vi "Write Dynamic.vi"(8 "error in (no error)":errorcluster, 10 "Dynamic data":dynamicdata(graph), 11 "tdms file":refnum<k34>) -> (0 "error out":errorcluster, 3 "tdms file out":refnum<k34>)   [LabVIEW 2015]
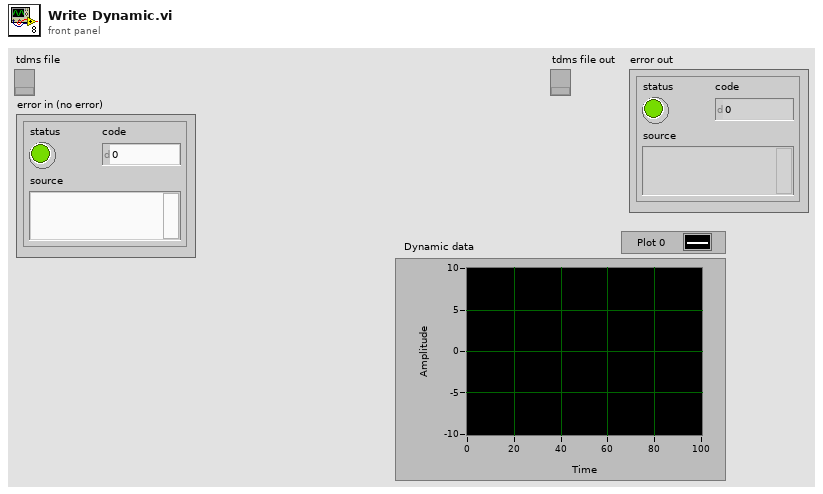
[diagram p1: front panel]
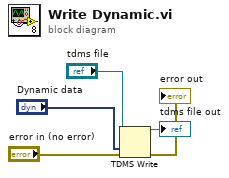
[diagram p0: block diagram]
diagram:
  n1 = TDMS Write(0:"tdms file", 9:"Dynamic data", 11:"error in (no error)") -> (4:→"tdms file out":refnum<k34>, 15:→"error out":errorcluster)  [unwired: 3 in, 2 out]
